vi "test_Add WaitSec Response.vi"(8 "error in (no error)":errorcluster, 11 "TestCase in":refnum<class "Instrument Addon Scripting API Messages Unit Tests.lvclass">) -> (0 "error out":errorcluster, 3 "TestCase out":refnum<class "Instrument Addon Scripting API Messages Unit Tests.lvclass">)   [LabVIEW 2018, in "Instrument Addon Scripting API Messages Unit Tests.lvclass"]
uses:
  Instrument Addon Scripting API Messages Unit Tests.lvclass
  APIs/Scripting API/TypeDefs/Linked Channel.ctl
  <vilib>/NI Veristand/Custom Device API/Custom Device Item Ref.ctl
  Addon/Addon Shared/Types/FG Control.ctl
  APIs/Scripting API/TypeDefs/Wait Response Settings.ctl
  Addon/Addon Shared/Types/Response Parameters.ctl
  Addon/Addon Shared/Types/Linked Channel Cluster.ctl
  Addon/Addon Shared/Types/Response Wait Type.ctl
  Addon/Addon Shared/SubVIs/Constants.vi
  <vilib>/NI/NI VeriStand Advanced SysDef API/_SubVIs/SysDef.Search.GUID.vi
  <vilib>/NI Veristand/Custom Device API/NI VeriStand - Get Item Property.vi
  <vilib>/NI Veristand/Custom Device API/Get Item Property (String).vi
  <vilib>/NI Veristand/Custom Device API/Get Item Property (String Array).vi
  <vilib>/NI Veristand/Custom Device API/Get Item Property (Double).vi
  <vilib>/NI Veristand/Custom Device API/Get Item Property (U32).vi
  <vilib>/NI Veristand/Custom Device API/Get Item Property (Boolean).vi
  <vilib>/NI Veristand/Custom Device API/NI VeriStand - Set Item Property.vi
  <vilib>/NI Veristand/Custom Device API/Set Item Property (String).vi
  <vilib>/NI Veristand/Custom Device API/Set Item Property (String Array).vi
  <vilib>/NI Veristand/Custom Device API/Set Item Property (Double).vi
  <vilib>/NI Veristand/Custom Device API/Set Item Property (U32).vi
  <vilib>/NI Veristand/Custom Device API/Set Item Property (Boolean).vi
  APIs/Scripting API/Messages/Add Response - Wait (sec).vi
  <vilib>/addons/_JKI Toolkits/VI Tester/TestCase.llb/TestCase.lvclass
  Instrument Addon Scripting API Test Assets/Instrument Addon Scripting API Test Assets.lvclass
  APIs/Scripting API/Instrument Addon Scripting API.lvlib
  <vilib>/NI Veristand/Custom Device API/Custom Device API.lvlib
  Addon/Addon Shared/Instrument Addon Shared.lvlib
  <vilib>/NI/NI VeriStand Advanced SysDef API/SysDef API/Advanced System Definition.lvlib
  C:/Program Files (x86)/National Instruments/LabVIEW 2018/vi.lib/addons/_JKI Toolkits/VI Tester/TestCase.llb/TestCase.lvclass
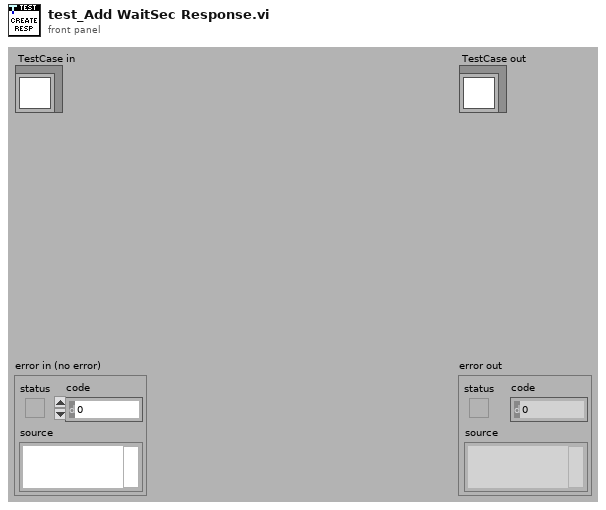
[diagram p1: front panel]
types:
  T1 = typedef "Instrument Addon Scripting API.lvlib/Wait Response Settings.ctl" = cluster{"Response Format":string, "Linked Channels":T2[], "Wait value (sec)":dbl, "Use Wait Channel":bool, "Channel Refnum":T3}
  T2 = typedef "Instrument Addon Scripting API.lvlib/Linked Channel.ctl" = cluster{"Variable Name":string, "Channel Refnum":T3}
  T3 = typedef "Custom Device API.lvlib/Custom Device Item Ref.ctl" = u64
  T4 = typedef "Instrument Addon Shared.lvlib/FG Control.ctl" = enum16{"Get", "Set"}
  T5 = typedef "Instrument Addon Shared.lvlib/Response Parameters.ctl" = cluster{"Response":string, "Linked Channels":T6[], "Type Value":dbl, "Wait Type":T7, "Use Channel":bool, "Channel Path":string}
  T6 = typedef "Instrument Addon Shared.lvlib/Linked Channel Cluster.ctl" = cluster{"Variable Name":string, "GUID":string}
  T7 = typedef "Instrument Addon Shared.lvlib/Response Wait Type.ctl" = enum16{"Byte Count", "Wait sec"}
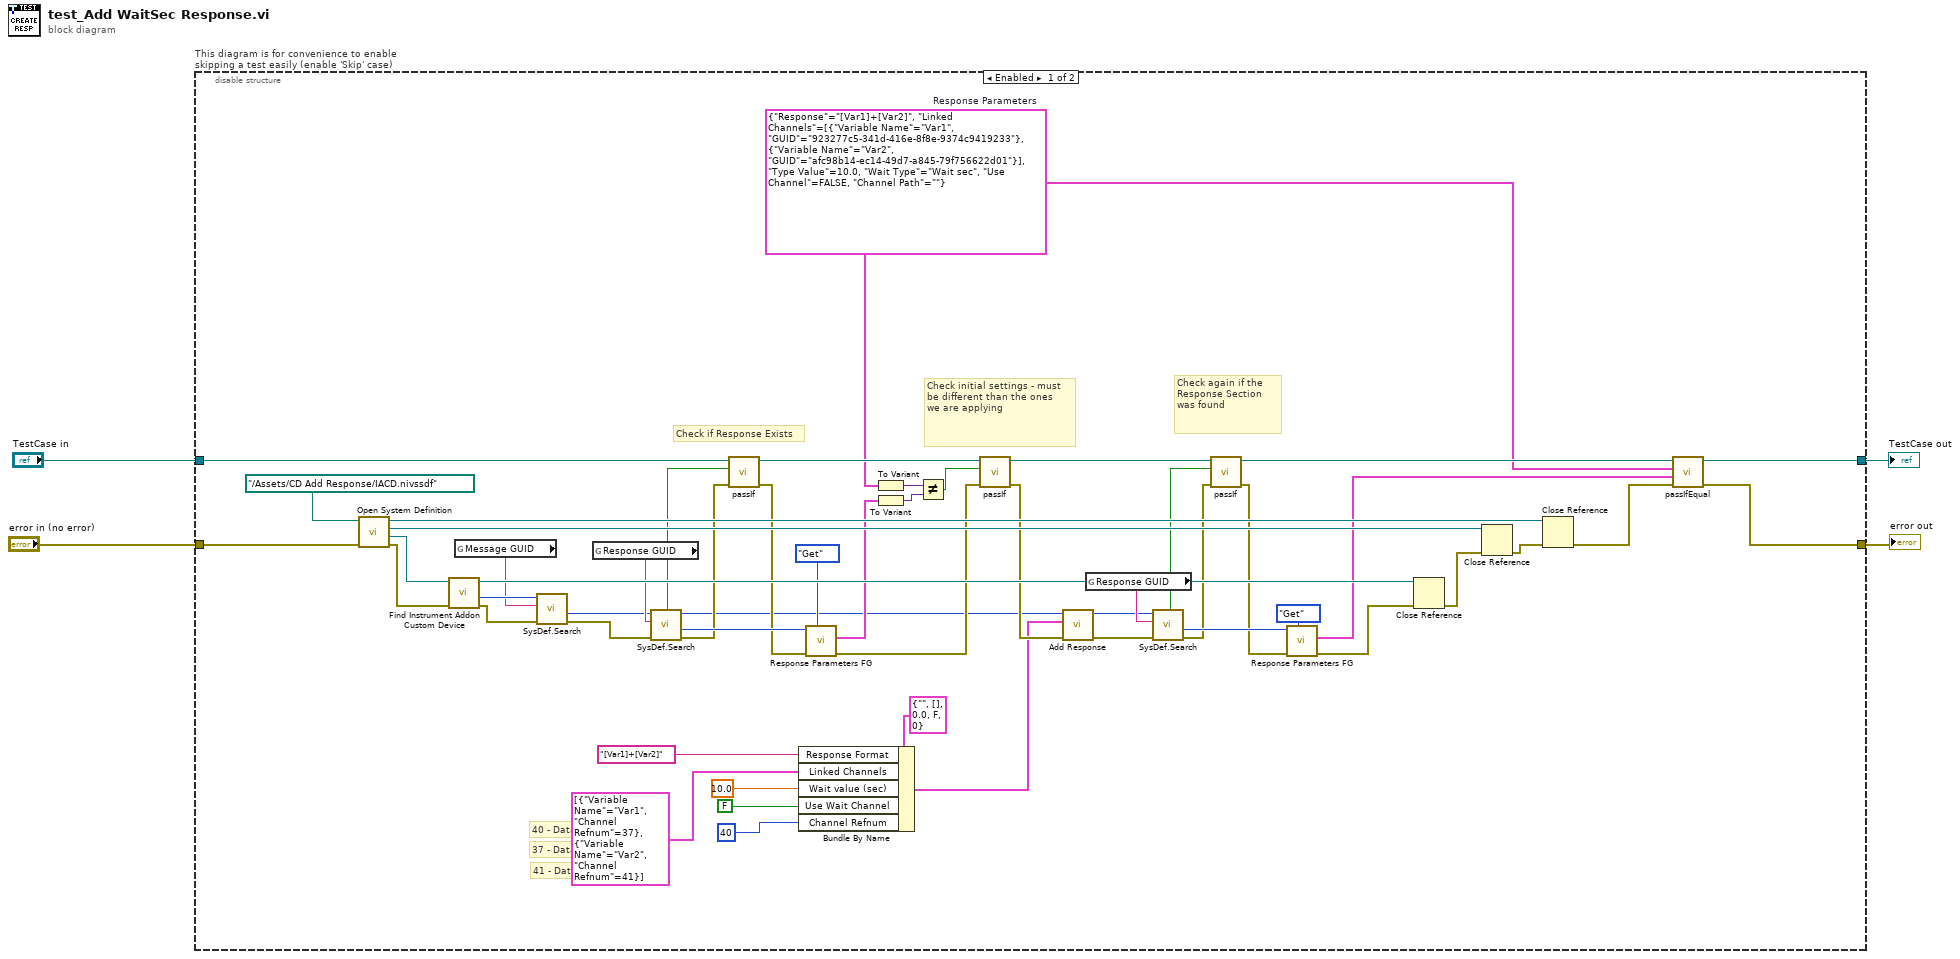
[diagram p0: block diagram]
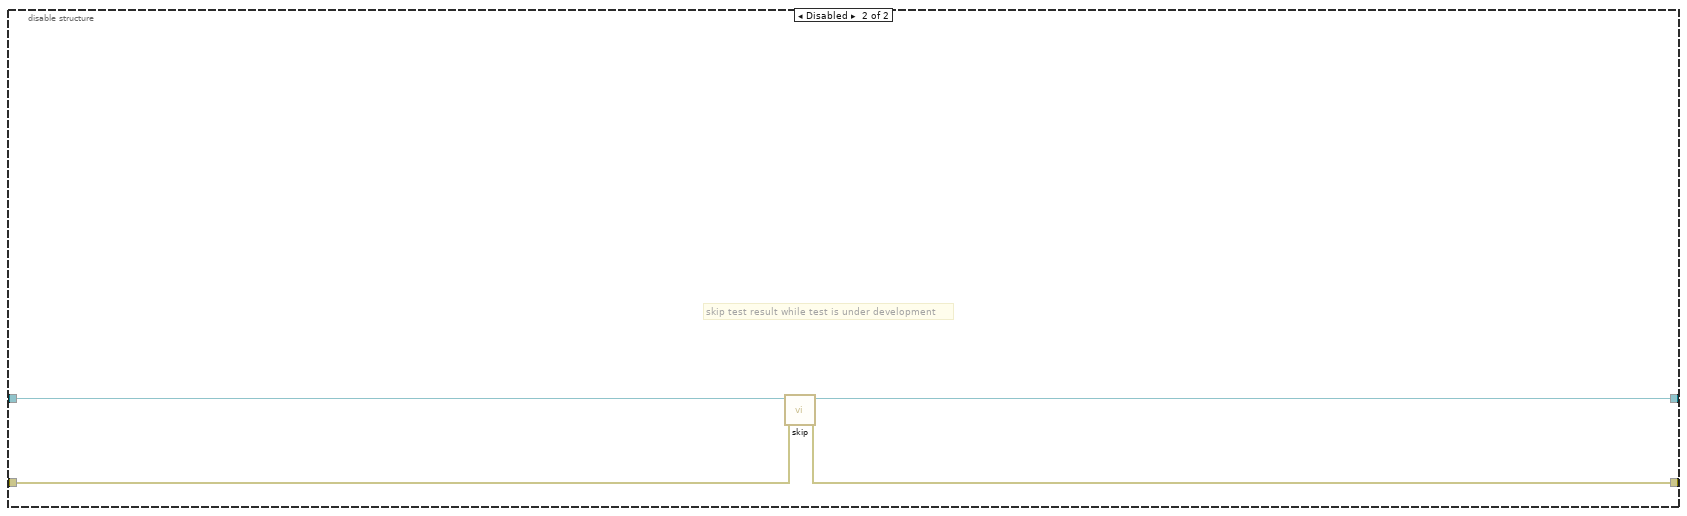
[diagram p2: hidden frame]
diagram:
  n1 = disable-structure "This diagram is for convenience to enable skipping a test easily (enable 'Skip' case)" shown="Enabled" {
    disable-tunnel: "TestCase in" -> [w26 w60]
    disable-tunnel: [w36 w58] -> w1
    disable-tunnel: [w35 w59] -> w3
    disable-tunnel: "error in (no error)" -> [w55 w57]
    frame Enabled {
      w5 = T5 {"Response"="[Var1]+[Var2]", "Linked Channels"=[{"Variable Name"="Var1", "GUID"="923277c5-341d-416e-8f8e-9374c9419233"}, {"Variable Name"="Var2", "GUID"="afc98b14-ec14-49d7-a845-79f756622d01"}], "Type Value"=10.0, "Wait Type"=enum."Wait sec", "Use Channel"=FALSE, "Channel Path"=""}  # Response Parameters
      # "Check again if the Response Section was found"
      # "Check initial settings - must be different than the ones\nwe are applying"
      # "Check if Response Exists"
      # "41 - Data 2"
      # "40 - Data 0"
      # "37 - Data 1"
      n2 = call "Open System Definition.vi"("error in (no error)"=w55, "System Definition File"=path "../Assets/CD Add Response/IACD.nivssdf" ("SDF file")) -> ("error out"=w53:errorcluster, "Target Refnum"=w52:refnum<k24>, "Root Refnum"=w51:refnum<k24>, "System Definition Refnum"=w39:refnum<k24>)  [unwired: 6 in]
      n3 = call "Find Instrument Addon Custom Device.vi"("error in"=w53, "target in"=w52) -> ("error out"=w9:errorcluster, "NodeID"=w10:u64, "target out"=w50:refnum<k24>)  [unwired: 7 in]
      n4 = global read "Constants.vi" "Message GUID"() -> (w8:string)
      n5 = call-poly <vilib>:"SysDef.Search.vi"("error in (no error)"=w9, "GUID"=w8, "nodeID"=w10) -> ("error out"=w7:errorcluster, "Value out"=w6:u64)  [unwired: 5 in, 2 out]
      n6 = global read "Constants.vi" "Response GUID"() -> (w32:string)
      n7 = call-poly <vilib>:"SysDef.Search.vi"("error in (no error)"=w7, "GUID"=w32, "nodeID"=w6) -> ("error out"=w24:errorcluster, "Value out"=w33:u64, "nodeID out"=w11:u64, "Found?"=w25:bool)  [unwired: 5 in]
      n8 = call-dynamic "passIf.vi"("error in (no error)"=w24, "pass"=w25, "TestCase in"=w26) -> ("error out"=w23:errorcluster, "TestCase out"=w22:refnum<class "Instrument Addon Scripting API Messages Unit Tests.lvclass">)  [unwired: 7 in]
      n9 = Bundle By Name(cluster=T1 {"Response Format"="", "Linked Channels"=[], "Wait value (sec)"=0.0, "Use Wait Channel"=FALSE, "Channel Refnum"=0} ("Settings"), "Response Format"="[Var1]+[Var2]", "Linked Channels"=T2[] [{"Variable Name"="Var1", "Channel Refnum"=37}, {"Variable Name"="Var2", "Channel Refnum"=41}], "Wait value (sec)"=10.0, "Use Wait Channel"=FALSE ("Use Byte Count channel"), "Channel Refnum"=T3 40) -> (w13:T1)
      n10 = call "Response Parameters FG.vi"("Action"=FG_Control."Get", "error in (no error)"=w23, "Item Ref in"=w33) -> ("error out"=w21:errorcluster, "Response Parameters"=w31:T5)  [unwired: 6 in, 1 out]
      n11 = To Variant(anything=w5) -> (Variant=w30:variant)
      n12 = To Variant(anything=w31) -> (Variant=w29:variant)
      n13 = Not Equal?(x=w30, y=w29) -> (x != y?=w28:bool)
      n14 = call-dynamic "passIf.vi"("error in (no error)"=w21, "pass"=w28, "TestCase in"=w22) -> ("error out"=w27:errorcluster, "TestCase out"=w20:refnum<class "Instrument Addon Scripting API Messages Unit Tests.lvclass">)  [unwired: 7 in]
      n15 = call-poly "Add Response.vi"("error in (no error)"=w27, "Settings"=w13, "Message in"=w11) -> ("error out"=w42:errorcluster, "Message out"=w41:T3)  [unwired: 7 in]
      n16 = global read "Constants.vi" "Response GUID"() -> (w43:string)
      n17 = call-poly <vilib>:"SysDef.Search.vi"("error in (no error)"=w42, "GUID"=w43, "nodeID"=w41) -> ("error out"=w19:errorcluster, "Value out"=w40:u64, "Found?"=w18:bool)  [unwired: 5 in, 1 out]
      n18 = call-dynamic "passIf.vi"("error in (no error)"=w19, "pass"=w18, "TestCase in"=w20) -> ("error out"=w17:errorcluster, "TestCase out"=w16:refnum<class "Instrument Addon Scripting API Messages Unit Tests.lvclass">)  [unwired: 7 in]
      n19 = call "Response Parameters FG.vi"("Action"=FG_Control."Get", "error in (no error)"=w17, "Item Ref in"=w40) -> ("error out"=w44:errorcluster, "Response Parameters"=w12:T5)  [unwired: 6 in, 1 out]
      n20 = Close Reference(reference=w50, error in (no error)=w44) -> (error out=w54:errorcluster)
      n21 = Close Reference(reference=w51, error in (no error)=w54) -> (error out=w38:errorcluster)
      n22 = Close Reference(reference=w39, error in (no error)=w38) -> (error out=w37:errorcluster)
      n23 = call-dynamic "passIfEqual.vi"("error in (no error)"=w37, "y"=w12, "x"=w5, "TestCase in"=w16) -> ("error out"=w35:errorcluster, "TestCase out"=w36:refnum<class "Instrument Addon Scripting API Messages Unit Tests.lvclass">)  [unwired: 6 in]
    }
    frame Disabled {
      # "skip test result while test is under development"
      n24 = call <vilib>:"skip.vi"("error in (no error)"=w57, "TestCase in"=w60) -> ("error out"=w59:errorcluster, "TestCase out"=w58:refnum<class "Instrument Addon Scripting API Messages Unit Tests.lvclass">)  [unwired: 8 in]
    }
  }
  "error out" <- w3
  "TestCase out" <- w1
